vi "GSP_F1_Global.vi"() -> ()   [LabVIEW 2015]
uses:
  SystemUtil/MotorStates.ctl
  SystemUtil/ThreadStates.ctl
panel:
  in  "Offset to 1st Pos Square":i32
  in  "Counts per Position Square":dbl=6222.17 format="%.2f"
  in  "F1_Name":string
  in  "F1 Thread State":T1
  in  "F1 Motor State":T2
  in  "F1 CPU Temp":dbl
  out "F1 Online":bool
  in  "Filter#":i32
  in  "Offset to 1st Pos":i32
  in  "Counts per Position":dbl=6222.17 format="%.2f"
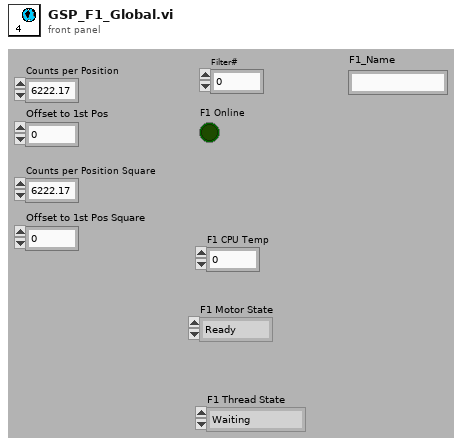
[diagram p1: front panel]
types:
  T1 = typedef "ThreadStates.ctl" = enum16{"Waiting", "Scripting", "Uninitialized", "Error"}
  T2 = typedef "MotorStates.ctl" = enum16{"Ready", "Moving", "Uninitialized", "Error"}
diagram:
